vi "SOUR_POW_DET_OBSOLETE.vi"(0 "VISA IN":refnum<visa-resource-name>, 1 "Internal or External Leveling":string, 5 "error in":errorcluster, 7 "Channel":i32) -> (14 "VISA Out":refnum<visa-resource-name>, 19 "error out":errorcluster)   [LabVIEW 2018, in "PNA-X.lvlib"]
doc: "SOURce<cnum>:POWer:DETector <char> OBSOLETE \n1828\n\n(Read-Write) The PNA models with external leveling are now OBSOLETE. \nSets the source leveling loop as Internal or External. \nParameters \n<cnum> Any existing channel number. If unspecified, value is set to 1 \n<char> INTernal - Internal leveling is applied to the source \nEXTernal - External leveling is applied to the source through a rear-panel \nconnector. ONLY provided on 3 GHz, 6 GHz, and 9 GHz PNA models. \nExamples SOUR:POW:DET INT \nsource2:power:detector external \nQuery Syntax SOURce<cnum>:POWer:DETector? \nReturn Type Character \nDefault INTernal"
uses:
  PNA-X.lvlib
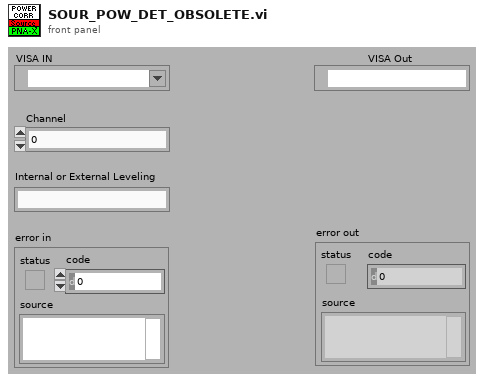
[diagram p1: front panel]
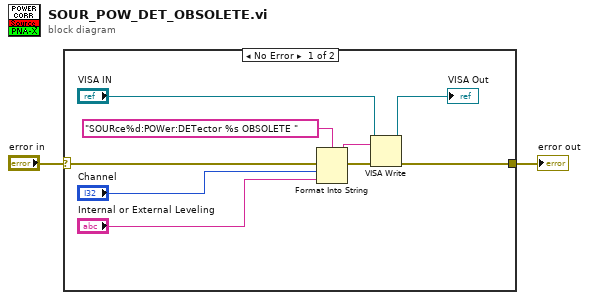
[diagram p0: block diagram]
diagram:
  n1 = case shown="No Error" "error in" {
    selector: "error in" -> [w11 w12]
    tunnel: [w6 w12] -> w1
    frame No Error {
      n2 = Format Into String(format string="SOURce%d:POWer:DETector %s OBSOLETE " ("Cmdline"), error in=w11, "Channel", "Internal or External Leveling") -> (resulting string=w9:string, error out=w10:errorcluster)  [unwired: 1 in]
      n3 = VISA Write(VISA resource name="VISA IN", write buffer=w9, error in (no error)=w10) -> (VISA resource name out=→"VISA Out":refnum<visa-resource-name>, error out=w6:errorcluster)  [unwired: 1 out]
    }
    frame Error {
    }
  }
  "error out" <- w1
